vi "face update.vi"(6 "slice number":u8, 7 "reverse? (F)":bool, 8 "error in (no error)":errorcluster, 9 "slice type":T1, 10 "slice":T2, 11 "face in":T3) -> (0 "error out":errorcluster, 3 "face out":T3)   [LabVIEW 2011]
uses:
  Typedef/face.ctl
  Typedef/slice.ctl
  Typedef/slice type.ctl
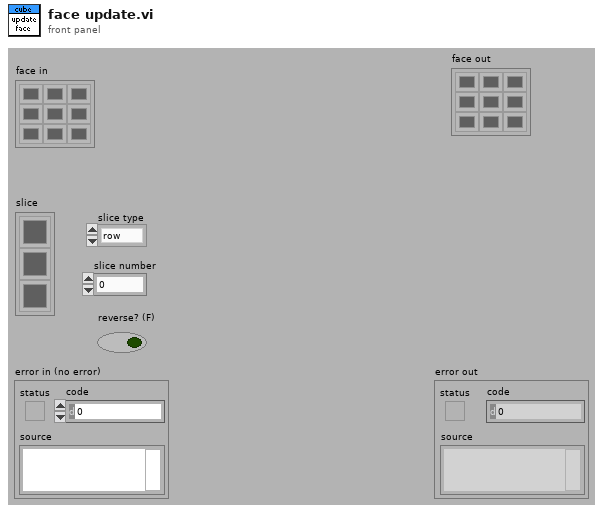
[diagram p1: front panel]
types:
  T1 = typedef "slice type.ctl" = enum16{"row", "col"}
  T2 = typedef "slice.ctl" = u32[]
  T3 = typedef "face.ctl" = u32[][]
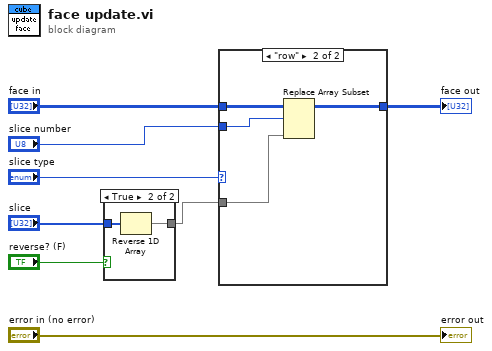
[diagram p0: block diagram]
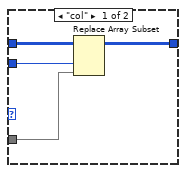
[diagram p3: hidden frame]
diagram:
  n1 = case shown="True" "reverse? (F)" {
    tunnel: "slice" -> [w9 w11]
    tunnel: [w9 w10] -> w1
    frame False {
    }
    frame True {
      n2 = Reverse 1D Array(array=w11) -> (reversed array=w10:T2)
    }
  }
  n3 = case shown="\"row\"" "slice type" {
    tunnel: "face in" -> [w15 w19]
    tunnel: "slice number" -> [w14 w16]
    tunnel: w1 -> [w13 w18]
    tunnel: [w12 w17] -> w6
    frame "col" {
      n4 = Replace Array Subset(array=w15, new element=w13, index (col)=w14) -> (w12:T3)  [unwired: 1 in]
    }
    frame "row" {
      n5 = Replace Array Subset(array=w19, new element=w18, index (row)=w16) -> (w17:T3)  [unwired: 1 in]
    }
  }
  "face out" <- w6
  "error out" <- "error in (no error)"
